vi "Variable G Script.vi"() -> ()   [LabVIEW 2010]
panel:
  in  "G Sizes":T1
  in  "Target Directory":path=path "D:/Ab-initio/VASP Calcs/2D_Grain Boundaries/Batch25_20130914"
  in  "Structure Name":string="A3B12_Lamallar"
  in  "Structure File":path=path "D:/Ab-initio/VASP Calcs/2D_Grain Boundaries/Batch18_20130828/A3B12_Periodic_Twin/CONTCAR"
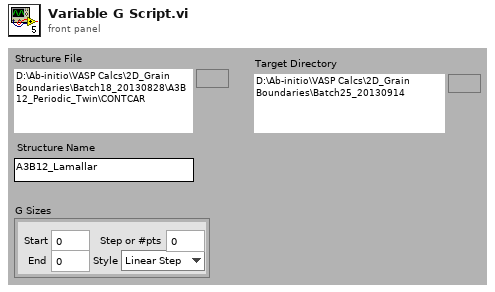
[diagram p1: front panel]
types:
  T1 = cluster{"Start":dbl, "End":dbl, "Step or #pts":dbl, "Style":enum16{"Linear Step", "Linear Pts", "Log Pts"}}
  T2 = cluster{"Structure Name":string, "Lattice vector a":dbl[], "Lattice vector b":dbl[], "Lattice vector c":dbl[], "Atoms Array":cluster{"Atom Name":string, "Positions (Direct)":dbl[][], "Positions (Cartesian)":dbl[][]}[], "# of atoms":i32}
  T3 = enum32{"Gamma Centered Monkhurst-Pack", "Monkhurst-Pack"}
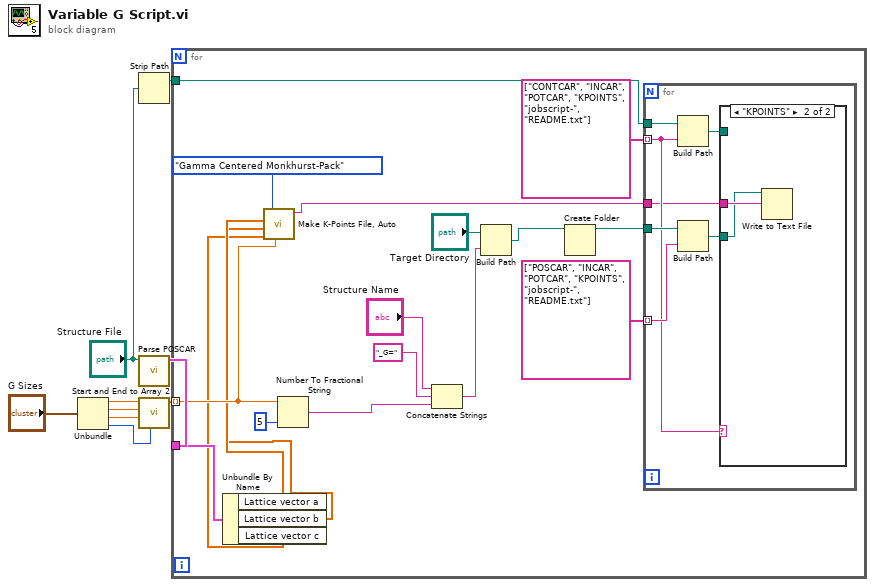
[diagram p0: block diagram]
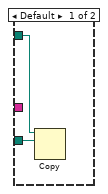
[diagram p2: hidden frame]
diagram:
  n1 = Unbundle("G Sizes") -> ("Start"=w7:dbl, "End"=w6:dbl, "Step or #pts"=w5:dbl, "Style"=w4:enum16{"Linear Step", "Linear Pts", "Log Pts"})
  n2 = Strip Path(path="Structure File") -> (stripped path=w1:path)  [unwired: 1 out]
  n3 = call "Parse POSCAR.vi"("POSCAR File"="Structure File") -> ("Structure"=w9:T2)  [unwired: 7 in, 3 out]
  n4 = call "Start and End to Array 2.vi"("Sweep Style"=w4, "Step or # Pts"=w5, "End"=w6, "Start"=w7) -> ("Array"=w3:dbl[])  [unwired: 7 in]
  n5 = for {
    tunnel: w9 -> [w23]
    tunnel: w3 -> [w15] mode=indexing
    tunnel: w1 -> [w18]
    n6 = Unbundle By Name(w23) -> ("Lattice vector a"=w14:dbl[], "Lattice vector b"=w13:dbl[], "Lattice vector c"=w12:dbl[])
    n7 = call "Make K-Points File, Auto.vi"("|G| Factor"=w15, "Lattice vector c"=w12, "Lattice vector b"=w13, "Lattice vector a"=w14, "Auto Type"=T3."Gamma Centered Monkhurst-Pack") -> ("K-Points File"=w10:string)  [unwired: 6 in]
    n8 = Number To Fractional String(number=w15, precision (6)=i16 5) -> (F-format string=w22:string)  [unwired: 2 in]
    n9 = Concatenate Strings("Structure Name", "_G=" ("string"), w22) -> (w24:string)
    n10 = Build Path(base path="Target Directory", name or relative path=w24) -> (appended path=w16:path)
    n11 = Create Folder(path (use dialog)=w16) -> (created path=w19:path)  [unwired: 2 in, 2 out]
    n12 = for {
      tunnel: w18 -> [w34]
      tunnel: w19 -> [w32]
      tunnel: string[] ["CONTCAR", "INCAR", "POTCAR", "KPOINTS", "jobscript-", "README.txt"] -> [w29] mode=indexing
      tunnel: string[] ["POSCAR", "INCAR", "POTCAR", "KPOINTS", "jobscript-", "README.txt"] -> [w30] mode=indexing
      tunnel: w10 -> [w28]
      n13 = Build Path(base path=w34, name or relative path=w29) -> (appended path=w33:path)
      n14 = Build Path(base path=w32, name or relative path=w30) -> (appended path=w31:path)
      n15 = case shown="\"KPOINTS\"" w29 {
        tunnel: w33 -> [w36 _]
        tunnel: w31 -> [w35 w37]
        tunnel: w28 -> [_ w38]
        frame Default {
          n16 = Copy(10:w35, 11:w36) -> ()  [unwired: 3 in, 3 out]
        }
        frame "KPOINTS" {
          n17 = Write to Text File(file (use dialog)=w37, text=w38) -> ()  [unwired: 2 in, 3 out]
        }
      }
    }
  }
